vi "Torque_measuring_device.vi"() -> ()   [LabVIEW 2026]
uses:
  <vilib>/Instr/_visa.llb/VISA Configure Serial Port (Instr).vi
  <vilib>/ptbypt/NI_PtbyPt.lvlib
panel:
  out "mean":dbl format="%0.2f"
  out "Torque. Nm":dbl(graph)
  out "Max_torque":dbl
  out "number":i32
  out "Electric_value":dbl(graph)
  in  "termination char\n(0xA = '\\n' = LF)":u8=10 format="%.0x"
  out "error out 2":errorcluster
  out "error out":errorcluster
  out "Numeric 2":i32
  out "Numeric":i32
  out "element":string
  out "read buffer":string
  in  "stop":bool
  in  "VISA resource name":refnum<visa-resource-name>
  in  "Enable Termination\nChar (T)":bool=TRUE
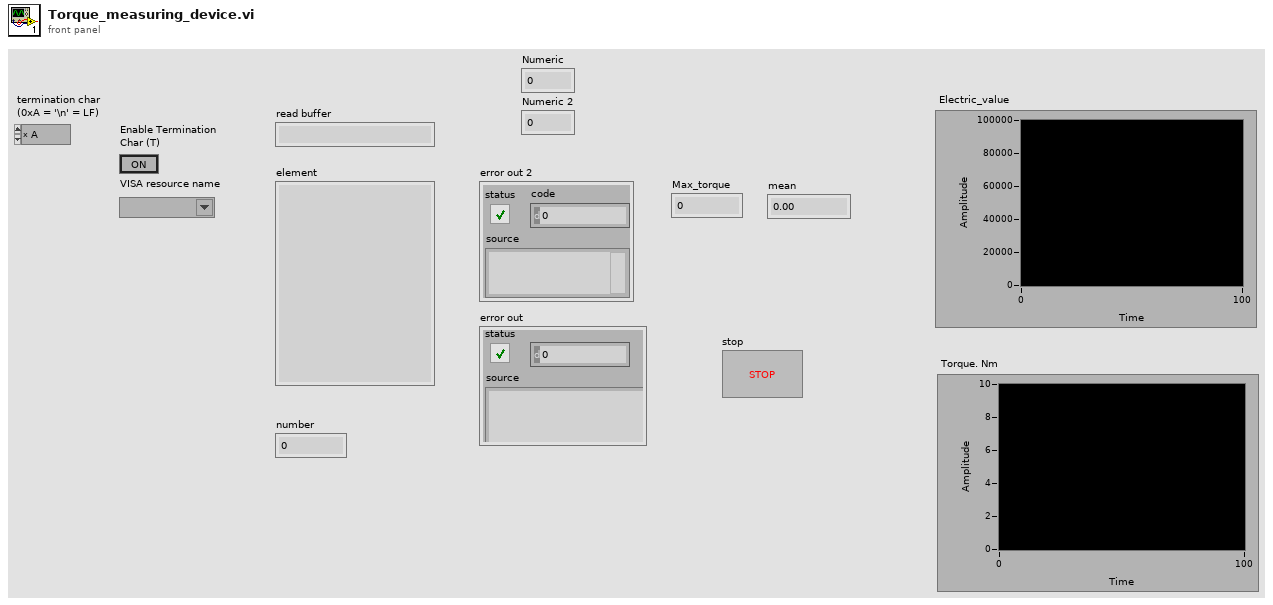
[diagram p1: front panel]
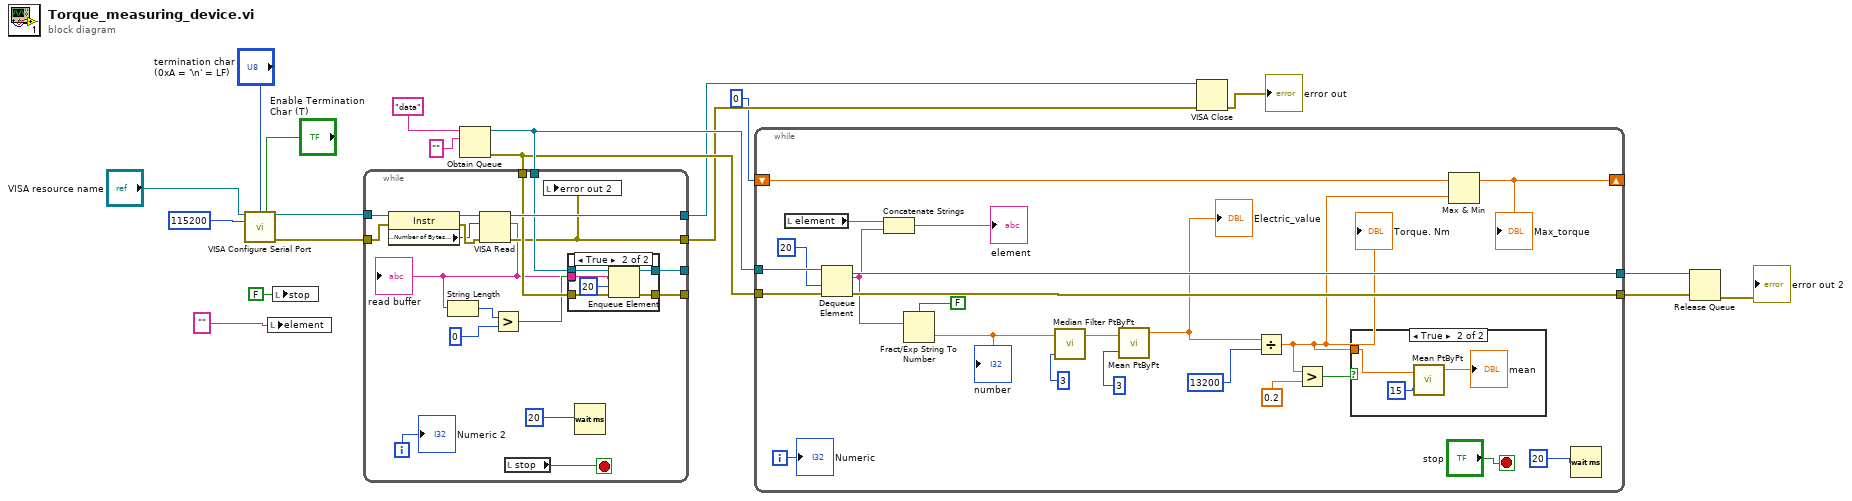
[diagram p0: block diagram]
diagram:
  n1 = call-poly "VISA Configure Serial Port"("VISA resource name"="VISA resource name", "termination char\n(0xA = '\\n' = LF)"="termination char\n(0xA = '\\n' = LF)", "Enable Termination\nChar (T)"="Enable Termination\nChar (T)", "baud rate (115200)"=u32 115200) -> ("VISA resource name out"=w14:refnum<visa-resource-name>, "error out"=w11:errorcluster)  [unwired: 10 in]
  n2 = local write "element"("" ("element")) -> ()
  n3 = local write "stop"(FALSE ("stop")) -> ()
  n4 = Obtain Queue(name (unnamed)="data", element data type="") -> (queue out=w13:refnum<queue>, error out=w12:errorcluster)  [unwired: 3 in, 1 out]
  n5 = while {
    tunnel: w14 -> [w31]
    tunnel: [w37] -> w5
    tunnel: w11 -> [w30]
    tunnel: [w27] -> w4
    tunnel: w13 -> [w35]
    tunnel: w12 -> [w34]
    tunnel: [w33] -> _
    tunnel: [w32] -> _
    i -> [w36]
    stop <- w25 stop-if-true
    n6 = property class="Instr"(reference=w31, error in=w30) -> (reference out=w28:refnum<visa-resource-name>, error out=w29:errorcluster, "Serial Settings:Number of Bytes at Serial Port"=w24:u32)
    n7 = VISA Read(VISA resource name=w28, byte count=w24, error in (no error)=w29) -> (VISA resource name out=w37:refnum<visa-resource-name>, read buffer=w20:string, error out=w27:errorcluster)  [unwired: 1 out]
    "read buffer" <- w20
    n8 = String Length(string=w20) -> (length=w23:i32)
    n9 = Greater?(x=w23, y=0 ("timeout in ms (-1)")) -> (0:w21:bool)
    n10 = local read "stop"() -> (w25:bool)
    n11 = local write "error out 2"(w27) -> ()
    n12 = case shown="True" w21 {
      tunnel: w35 -> [w38 w45]
      tunnel: w34 -> [w39 w44]
      tunnel: [w38 w43] -> w33
      tunnel: [w39 w42] -> w32
      tunnel: w20 -> [_ w40]
      frame False {
      }
      frame True {
        n13 = Enqueue Element(queue=w45, element=w40, timeout in ms (-1)=20, error in (no error)=w44) -> (queue out=w43:refnum<queue>, error out=w42:errorcluster)  [unwired: 1 out]
      }
    }
    n14 = Wait (ms)(milliseconds to wait=u32 20) -> ()  [unwired: 1 out]
    "Numeric 2" <- w36
  }
  n15 = while {
    tunnel: w13 -> [w67]
    tunnel: w12 -> [w66]
    tunnel: [w65] -> w10
    tunnel: [w64] -> w9
    shift-right: [w57] -> _
    shift-left: 0 ("timeout in ms (-1)") -> [w58]
    i -> [w63]
    stop <- "stop" stop-if-true
    n16 = local read "element"() -> (w61:string)
    n17 = Dequeue Element(queue=w67, timeout in ms (-1)=20, error in (no error)=w66) -> (queue out=w64:refnum<queue>, element=w51:string, error out=w65:errorcluster)  [unwired: 1 out]
    n18 = Concatenate Strings(w61, w51) -> (→"element":string)
    n19 = Fract/Exp String To Number(use system decimal point (T)=FALSE, string=w51) -> (number=w50:dbl)  [unwired: 2 in, 1 out]
    "number" <- w50
    n20 = call <vilib>:"Median Filter PtByPt.vi"("rank"=3, "x"=w50) -> ("Filtered x"=w55:dbl)  [unwired: 2 in, 1 out]
    n21 = call <vilib>:"Mean PtByPt.vi"("x"=w55, "sample length"=3) -> ("mean"=w53:dbl)  [unwired: 2 in, 1 out]
    "Electric_value" <- w53
    n22 = Divide(x=w53, y=13200 ("sample length")) -> (x/y=w46:dbl)
    "Torque. Nm" <- w46
    n23 = Greater?(x=w46, y=0.2) -> (0:w47:bool)
    n24 = case shown="True" w47 {
      tunnel: w46 -> [_ w71]
      frame False {
      }
      frame True {
        n25 = call <vilib>:"Mean PtByPt.vi"("x"=w71, "sample length"=15) -> ("mean"=→"mean":dbl)  [unwired: 2 in, 1 out]
      }
    }
    n26 = Max & Min(x=w58, y=w46) -> (max(x,y)=w57:dbl)  [unwired: 1 out]
    "Max_torque" <- w57
    n27 = Wait (ms)(milliseconds to wait=u32 20) -> ()  [unwired: 1 out]
    "Numeric" <- w63
  }
  n28 = VISA Close(VISA resource name=w5, error in (no error)=w4) -> (error out=→"error out":errorcluster)
  n29 = Release Queue(queue=w9, error in (no error)=w10) -> (error out=→"error out 2":errorcluster)  [unwired: 1 in, 2 out]
